vi "Controller.vi"(5 "PID gain schedule":T1(array[cluster])=[{"PID gains"={"proportional gain (Kc)"=1.0, "integral time (Ti, min)"=0.01, "derivative time (Td, min)"=0.0}, "max value"=100.0}] {"max value" format="%.2f"; "PID gains"."derivative time (Td, min)" format="%.6f"; "PID gains"."integral time (Ti, min)" format="%.6f"; "PID gains"."proportional gain (Kc)" format="%.6f"}, 6 "error in (no error)":errorcluster, 7 "setpoint profile":cluster{"time (s)":dbl, "setpoint":dbl}[](array[cluster]), 8 "Gain Schedule Table Path":path, 9 "Process_REF":string="Temperature") -> (0 "error out":errorcluster)   [LabVIEW 2018]
uses:
  <vilib>/addons/control/pid/pid.llb/PID Gain Schedule (DBL).vi
  <vilib>/addons/control/pid/pid.llb/PID Advanced (DBL).vi
  <vilib>/addons/control/pid/NI_PID_pid.lvlib
panel:
  in  "Reinitialize Profile":bool
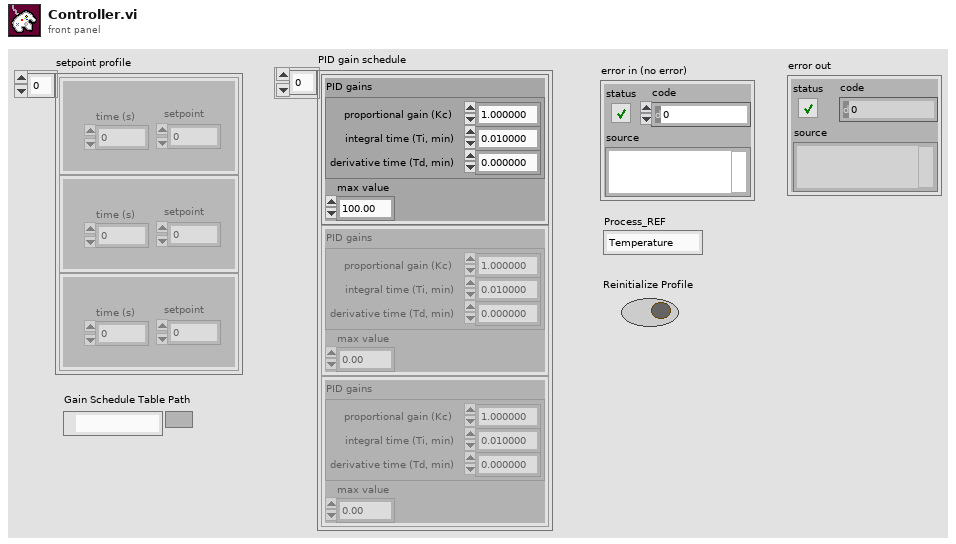
[diagram p1: front panel]
types:
  T1 = cluster{"PID gains":cluster{"proportional gain (Kc)":dbl, "integral time (Ti, min)":dbl, "derivative time (Td, min)":dbl}, "max value":dbl}[]
  T2 = cluster{"proportional gain (Kc)":dbl, "integral time (Ti, min)":dbl, "derivative time (Td, min)":dbl}
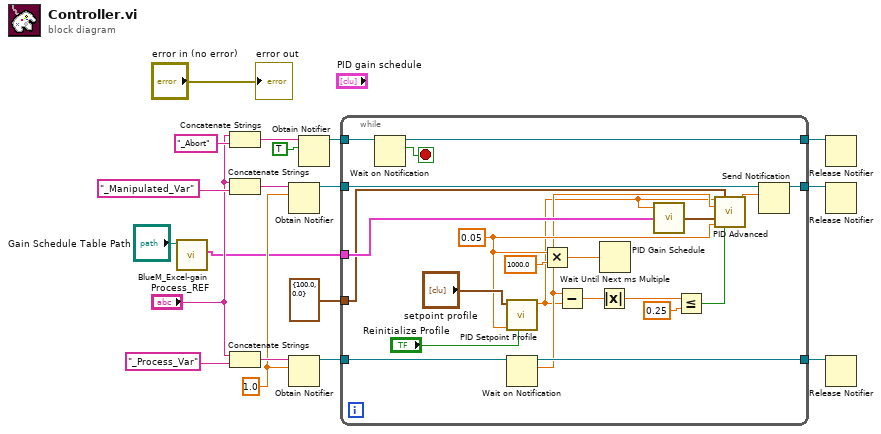
[diagram p0: block diagram]
diagram:
  w8 = 1.0
  n1 = call "BlueM_Excel-gain.vi"("file path (use dialog)"="Gain Schedule Table Path") -> ("PID gain schedule"=w1:T1)  [unwired: 10 in]
  n2 = Concatenate Strings("Process_REF", "_Abort") -> (w13:string)
  n3 = Concatenate Strings("Process_REF", "_Manipulated_Var" ("string")) -> (w11:string)
  n4 = Concatenate Strings("Process_REF", "_Process_Var") -> (w9:string)
  n5 = Obtain Notifier(name (unnamed)=w11, notification data type=w8) -> (notifier out=w10:refnum<notifier>)  [unwired: 2 in, 2 out]
  n6 = Obtain Notifier(name (unnamed)=w9, notification data type=w8) -> (notifier out=w7:refnum<notifier>)  [unwired: 2 in, 2 out]
  n7 = Obtain Notifier(name (unnamed)=w13, notification data type=TRUE) -> (notifier out=w12:refnum<notifier>)  [unwired: 2 in, 2 out]
  n8 = while {
    tunnel: w1 -> [w40]
    tunnel: w7 -> [w23]
    tunnel: w12 -> [w27]
    tunnel: [w25] -> w15
    tunnel: [w28] -> w6
    tunnel: w10 -> [w29]
    tunnel: [w30] -> w16
    tunnel: cluster{"output high":dbl, "output low":dbl} {"output high"=100.0, "output low"=0.0} ("output range") -> [w22]
    stop <- w26 stop-if-true
    w31 = 0.05
    n9 = Wait on Notification(notifier=w27) -> (notifier out=w28:refnum<notifier>, notification=w26:bool)  [unwired: 3 in, 2 out]
    n10 = call <vilib>:"PID Setpoint Profile.vi"("reinitialize? (F)"="Reinitialize Profile", "dt (s)"=w31, "setpoint profile"="setpoint profile") -> ("setpoint"=w21:dbl)  [unwired: 3 in, 3 out]
    n11 = Wait on Notification(notifier=w23) -> (notifier out=w25:refnum<notifier>, notification=w24:dbl)  [unwired: 3 in, 2 out]
    n12 = Multiply(x=w31, y=1000.0) -> (x*y=w38:dbl)
    n13 = Subtract(x=w24, y=w21) -> (x-y=w36:dbl)
    n14 = Absolute Value(x=w36) -> (abs(x)=w35:dbl)
    n15 = Wait Until Next ms Multiple(millisecond multiple=w38) -> ()  [unwired: 1 out]
    n16 = call-poly <vilib>:"PID Gain Schedule.vi"("PID gain schedule"=w40, "gain scheduling value"=w21) -> ("PID gains out"=w41:T2)  [unwired: 2 in, 1 out]
    n17 = Less Or Equal?(x=w35, y=0.25) -> (x <= y?=w33:bool)
    n18 = call-poly <vilib>:"PID Advanced.vi"("setpoint"=w21, "output range"=w22, "process variable"=w24, "PID gains"=w41, "dt (s)"=w31, "reinitialize? (F)"=w33) -> ("output"=w20:dbl)  [unwired: 8 in, 1 out]
    n19 = Send Notification(notification=w20, notifier=w29) -> (notifier out=w30:refnum<notifier>)  [unwired: 1 in, 1 out]
  }
  n20 = Release Notifier(notifier=w6) -> ()  [unwired: 2 in, 3 out]
  n21 = Release Notifier(notifier=w16) -> ()  [unwired: 2 in, 3 out]
  n22 = Release Notifier(notifier=w15) -> ()  [unwired: 2 in, 3 out]
  "error out" <- "error in (no error)"
